vi "checkBeginZigZagPlay.vi"(8 "error in (no error)":errorcluster, 10 "Game":refnum<class "Game.lvclass">, 11 "ZigZagPlay in":refnum<class "ZigZagPlay.lvclass">) -> (0 "error out":errorcluster, 2 "TestMode":bool, 3 "ZigZagPlay out":refnum<class "ZigZagPlay.lvclass">)   [LabVIEW 2023, in "ZigZagPlay.lvclass"]
uses:
  ZigZagPlay.lvclass
  Game_class/Game.lvclass
  Referee_class/command_interpreted.ctl
  Game_class/Game.lvclass/Game.ctl
  Referee_class/Referee.lvclass/Referee.ctl
  Game_class/Read TestMode.vi
  Game_class/Read Referee.vi
  Referee_class/Read command_interpreted.vi
  Referee_class/Referee.lvclass
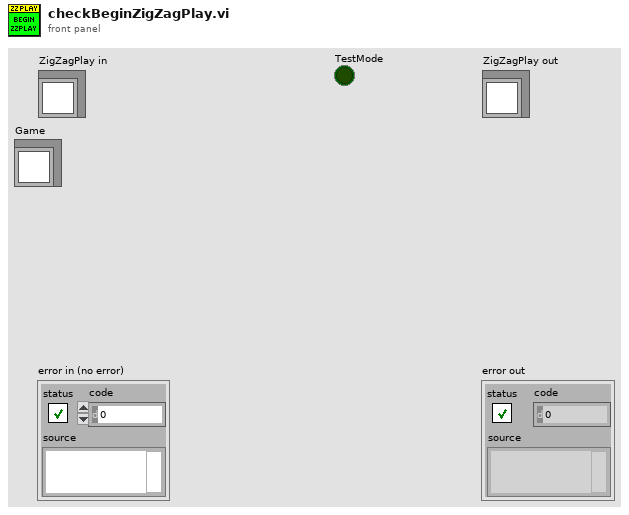
[diagram p1: front panel]
types:
  T1 = typedef "command_interpreted.ctl" = enum16{"Goal Ally", "Goal Enemy", "Ball Placement Enemy", "Ball Placement Ally", "Normal Half Time", "Extra Time  Break", "Extra Half Time", "None", "Post Game", "PKA Normal Start", "Prepare Kickoff Ally", "PKE Normal Start", "Prepare Kickoff Enemy", "Force Start", "Halt", "Timeout", "Prepare Penalty Ally", "Prepare Penalty Enemy", "PPA NormalStart", "PPE Normal Start", "Indirect Free Ally", "Direct Free Enemy", "Direct Free Ally", "Indirect Free Enemy", "Stop"}
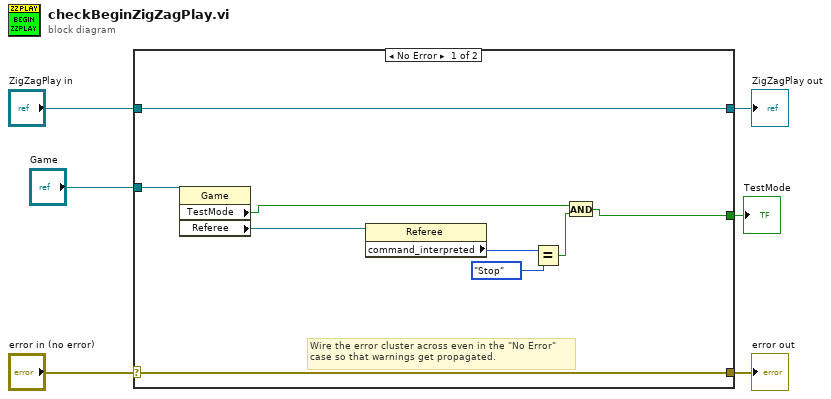
[diagram p0: block diagram]
diagram:
  n1 = case shown="No Error" "error in (no error)" {
    selector: "error in (no error)" -> [w14 w17]
    tunnel: [w14 w17] -> w5
    tunnel: [w15 w16] -> w3
    tunnel: "ZigZagPlay in" -> [w15 w16]
    tunnel: "Game" -> [w13 _]
    tunnel: [w7 _] -> w1
    frame No Error {
      # "Wire the error cluster across even in the \"No Error\"\ncase so that warnings get propagated."
      n2 = property class="Game"(reference=w13) -> ("TestMode"=w8:bool, "Referee"=w9:refnum<class "Referee.lvclass">)  [unwired: 1 in, 2 out]
      n3 = property class="Referee"(reference=w9) -> ("command_interpreted"=w12:T1)  [unwired: 1 in, 2 out]
      n4 = Equal?(x=w12, y=command_interpreted."Stop") -> (x = y?=w11:bool)
      n5 = And(x=w8, y=w11) -> (x .and. y?=w7:bool)
    }
    frame Error {
    }
  }
  "error out" <- w5
  "ZigZagPlay out" <- w3
  "TestMode" <- w1
